vi "GetType.vi"(8 "error in (no error)":errorcluster, 11 "Send Software Trigger [TRG] Msg":refnum<class "Send Software Trigger [TRG] Msg.lvclass">) -> (0 "error out":errorcluster, 2 "Data Sample":variant, 3 "Send Software Trigger [TRG] Msg":refnum<class "Send Software Trigger [TRG] Msg.lvclass">)   [LabVIEW 2015, in "CS++Fgen.lvlib" / "Send Software Trigger [TRG] Msg.lvclass"]
doc: "This VI delivers a sample of the data type format the message expects."
uses:
  Send Software Trigger [TRG] Msg.lvclass
  Send Software Trigger [TRG] Msg.lvclass/Send Software Trigger [TRG] Msg.ctl
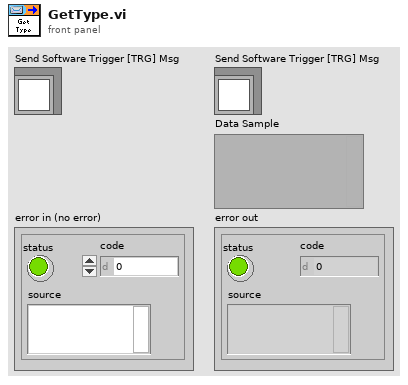
[diagram p1: front panel]
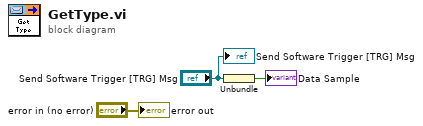
[diagram p0: block diagram]
diagram:
  n1 = Unbundle("Send Software Trigger [TRG] Msg") -> (→"Data Sample":bool)
  "error out" <- "error in (no error)"
  "Send Software Trigger [TRG] Msg" <- "Send Software Trigger [TRG] Msg"
